vi "Play Cine from File.vi"() -> ()   [LabVIEW 2013]
doc: "This example VI demonstrates how to acquire and display captured images stored in the internal RAM of a Phantom Camera using the Vision Research Phantom Series LabVIEW Driver."
uses:
  _Type Defs/PhFile InfName.ctl
  _Type Defs/PHCon IMRANGE.ctl
  _Type Defs/PhInt PhProcessImage Selectors.ctl
  VRI.lvlib
panel:
  in  "Delay (ms)":u32=100
  in  "szFileName":path
  in  "fGain16_8":dbl=1.0
  in  "Stop":bool
  out "Image Count":u32
  out "first image number":i32
  out "Current Image #":i32
  out "Preview":picture
  out "Error Out":errorcluster
  in  "error in (no error)":errorcluster
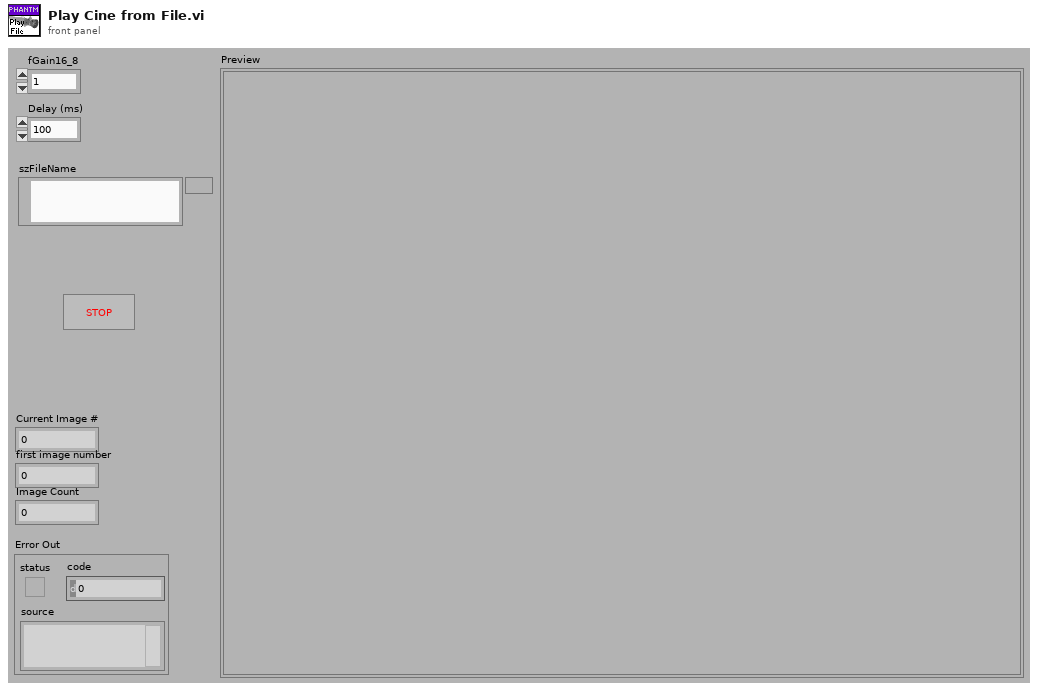
[diagram p1: front panel]
types:
  T1 = typedef "VRI.lvlib/PHCon IMRANGE.ctl" = cluster{"First":i32, "Cnt":u32}
  T2 = typedef "VRI.lvlib/PhFile InfName.ctl" = u32
  T3 = typedef "VRI.lvlib/PhInt PhProcessImage Selectors.ctl" = u16
  T4 = typedef "VRI.lvlib/PhInt IH.ctl" = cluster{"biSize":u32, "biWidth":i32, "biHeight":i32, "biPlanes":u16, "biBitCount":u16, "biCompresssion":u32, "biSizeImage":u32, "biXPelsPerMeter":i32, "biYPelsPerMeter":i32, "biClrUsed":u32, "biClrImportant":u32, "BlackLevel":i32, "WhiteLevel":i32}
  T5 = typedef "VRI.lvlib/BITMAPINFOHEADER.ctl" = cluster{"biSize":u32, "biWidth":i32, "biHeight":i32, "biPlanes":u16, "biBitCount":u16, "biCompression":u32, "biSizeImage":u32, "biXPelsPerMeter":i32, "biYPelsPerMeter":i32, "biClrUsed":u32, "biClrImportant":u32}
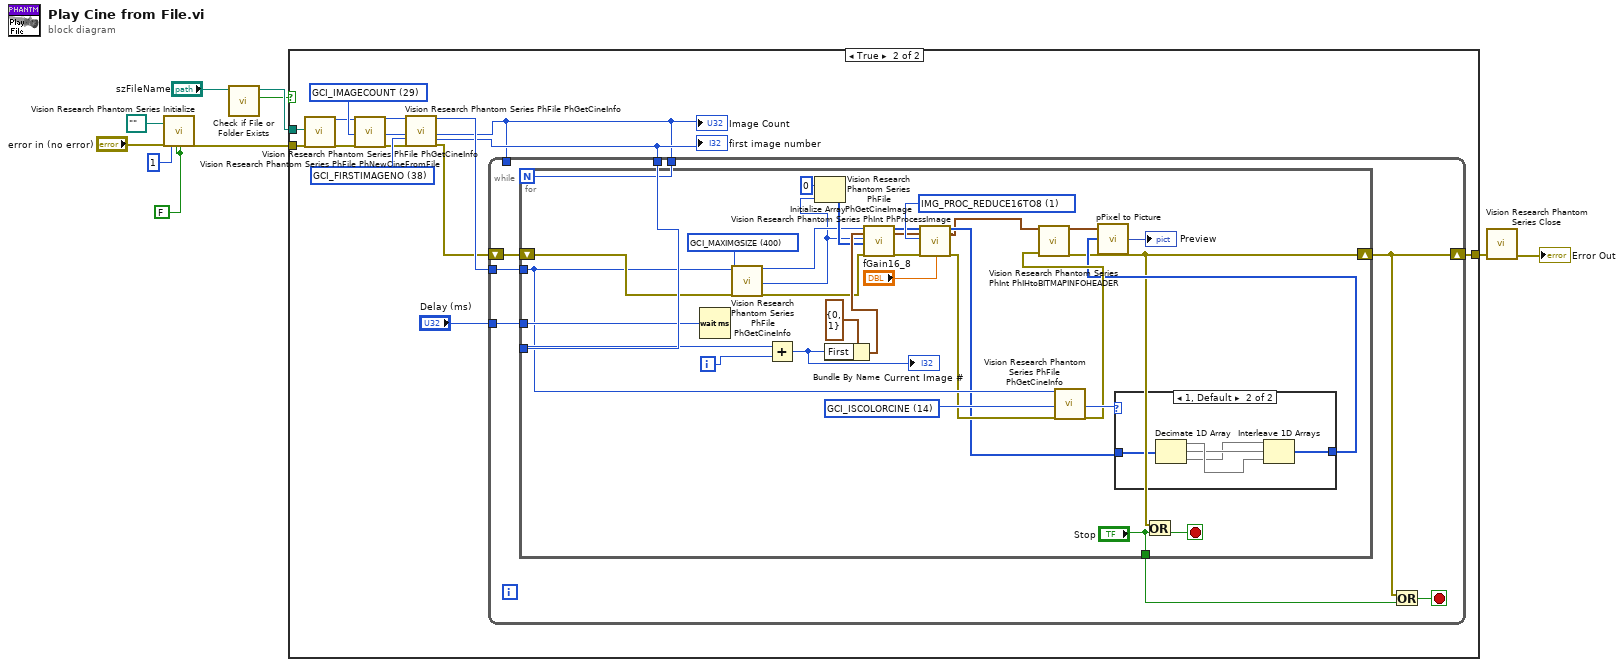
[diagram p0: block diagram]
diagram:
  w7 = FALSE ("ID Query (T: Check)")
  n1 = call "Vision Research Phantom Series Initialize.vi"("Storage Path (\"\")"=path "" ("Storage Path (\"\")"), "error in (no error)"="error in (no error)", "CallID"=u32 1, "ID Query (T: Check)"=w7, "Reset (F: Don't Reset)"=w7) -> ("Error Out"=w4:errorcluster)  [unwired: 14 out]
  n2 = call <vilib>:"Check if File or Folder Exists.vi"("path"="szFileName") -> ("file or folder exists?"=w1:bool, "dup path"=w2:path)  [unwired: 8 in, 1 out]
  n3 = case shown="True" w1 {
    tunnel: [w11 w25] -> w6
    tunnel: w2 -> [_ w24]
    tunnel: w4 -> [w11 w22]
    frame False {
    }
    frame True {
      w18 = T2 38 items=["GCI_CFA"=0, "GCI_FRAMERATE"=1, "GCI_EXPOSURE"=2, "GCI_AUTOEXPOSURE"=3, "GCI_REALBPP"=4, "GCI_CAMERASERIAL"=5, "GCI_HEADSERIAL0"=6, "GCI_HEADSERIAL1"=7, "GCI_HEADSERIAL2"=8, "GCI_HEADSERIAL3"=9, "GCI_TRIGTIMESEC"=10, "GCI_TRIGTIMEFR"=11, "GCI_ISFILECINE"=12, "GCI_IS16BPPCINE"=13, "GCI_ISCOLORCINE"=14, "GCI_ISMULTIHEADCINE"=15, "GCI_EXPOSURENS"=16, "GCI_EDREXPOSURENS"=17, "GCI_FRAMEDELAYNS"=19, "GCI_FROMFILETYPE"=20, "GCI_COMPRESSION"=21, "GCI_CAMERAVERSION"=22, "GCI_ROTATE"=23, "GCI_IMWIDTH"=24, "GCI_IMHEIGHT"=25, "GCI_IMWIDTHACQ"=26, "GCI_IMHEIGHTACQ"=27, "GCI_POSTTRIGGER"=28, "GCI_IMAGECOUNT"=29, "GCI_TOTALIMAGECOUNT"=30, "GCI_TRIGFRAME"=31, "GCI_AUTOEXPLEVEL"=32, "GCI_AUTOEXPTOP"=33, "GCI_AUTOEXPLEFT"=34, "GCI_AUTOEXPBOTTOM"=35, "GCI_AUTOEXPRIGHT"=36, "GCI_RECORDINGTIMEZONE"=37, "GCI_FIRSTIMAGENO"=38, "GCI_FIRSTMOVIEIMAGE"=39, "GCI_CINENAME"=40, "GCI_FRPSTEPS"=100, "GCI_FRP1X"=101, "GCI_FRP1Y"=102, "GCI_FRP2X"=103, "GCI_FRP2Y"=104, "GCI_FRP3X"=105, "GCI_FRP3Y"=106, "GCI_FRP4X"=107, "GCI_FRP4Y"=108, "GCI_WRITEERR"=109, "GCI_LENSDESCRIPTION"=110, "GCI_LENSAPERATURE"=111, "GCI_LENSFOCALLENGTH"=112, "GCI_WB"=200, "GCI_WBVIEW"=201, "GCI_BRIGHT"=202, "GCI_CONTRAST"=203, "GCI_GAMMA"=204, "GCI_GAMMAR"=223, "GCI_GAMMAB"=224, "GCI_SATURATION"=205, "GCI_HUE"=206, "GCI_FLIPH"=207, "GCI_FLIPV"=208, "GCI_FILTERCODE"=209, "GCI_IMFILTER"=210, "GCI_INTALGO"=211, "GCI_PEDESTALR"=212, "GCI_PEDESTALG"=213, "GCI_PEDESTALB"=214, "GCI_FLARE"=225, "GCI_CHROMA"=226, "GCI_TONE"=227, "GCI_ENABLEMATRICES"=228, "GCI_USERMATRIX"=229, "GCI_RESAMPLEACTIVE"=215, "GCI_RESAMPLEWIDTH"=216, "GCI_RESAMPLEHEIGHT"=217, "GCI_CROPACTIVE"=218, "GCI_CROPRECTANGLE"=219, "GCI_OFFSET16_8"=220, "GCI_GAIN16_8"=221, "GCI_DEMOSAICINGFUNCPTR"=222, "GCI_VFLIPVIEWACTIVE"=300, "GCI_MAXIMGSIZE"=400, "GCI_FRPIMGNOARRAY"=450, "GCI_FRPRATEARRAY"=451, "GCI_FRPSHAPEARRAY"=452, "GCI_TRIGTC"=470, "GCI_TRIGTCU"=471, "GCI_PBRATE"=472, "GCI_TCRATE"=473, "GCI_SAVERANGE"=500, "GCI_SAVEFILENAME"=501, "GCI_SAVEFILETYPE"=502, "GCI_SAVE16BIT"=503, "GCI_SAVEPACKED"=504, "GCI_SAVEXML"=505, "GCI_SAVESTAMPTIME"=506, "GCI_SAVEAVIFRAMERATE"=520, "GCI_SAVEAVICOMPRESSORLIST"=521, "GCI_SAVEAVICOMPRESSORINDEX"=522, "GCI_SAVEDPXLSB"=530, "GCI_SAVEDPXTO10BPS"=531, "GCI_SAVEDPXDATAPACKING"=532, "GCI_SAVEDPX10BITLOG"=533, "GCI_SAVEDPXEXPORTLOGLUT"=534, "GCI_SAVEDPX10BITLOGREFWHITE"=535, "GCI_SAVEDPX10BITLOGREFBLACK"=536, "GCI_SAVEDPX10BITLOGGAMMA"=537, "GCI_SAVEDPX10BITLOGFILMGAMMA"=538, "GCI_SAVEQTPLAYBACKRATE"=550, "GCI_SAVECCIQUALITY"=560, "GCI_UNCALIBRATEDIMAGE"=600, "GCI_NOPROCESSING"=601, "GCI_BADPIXELREPAIR"=602] ("InfName")
      w21 = T2 29 items=["GCI_CFA"=0, "GCI_FRAMERATE"=1, "GCI_EXPOSURE"=2, "GCI_AUTOEXPOSURE"=3, "GCI_REALBPP"=4, "GCI_CAMERASERIAL"=5, "GCI_HEADSERIAL0"=6, "GCI_HEADSERIAL1"=7, "GCI_HEADSERIAL2"=8, "GCI_HEADSERIAL3"=9, "GCI_TRIGTIMESEC"=10, "GCI_TRIGTIMEFR"=11, "GCI_ISFILECINE"=12, "GCI_IS16BPPCINE"=13, "GCI_ISCOLORCINE"=14, "GCI_ISMULTIHEADCINE"=15, "GCI_EXPOSURENS"=16, "GCI_EDREXPOSURENS"=17, "GCI_FRAMEDELAYNS"=19, "GCI_FROMFILETYPE"=20, "GCI_COMPRESSION"=21, "GCI_CAMERAVERSION"=22, "GCI_ROTATE"=23, "GCI_IMWIDTH"=24, "GCI_IMHEIGHT"=25, "GCI_IMWIDTHACQ"=26, "GCI_IMHEIGHTACQ"=27, "GCI_POSTTRIGGER"=28, "GCI_IMAGECOUNT"=29, "GCI_TOTALIMAGECOUNT"=30, "GCI_TRIGFRAME"=31, "GCI_AUTOEXPLEVEL"=32, "GCI_AUTOEXPTOP"=33, "GCI_AUTOEXPLEFT"=34, "GCI_AUTOEXPBOTTOM"=35, "GCI_AUTOEXPRIGHT"=36, "GCI_RECORDINGTIMEZONE"=37, "GCI_FIRSTIMAGENO"=38, "GCI_FIRSTMOVIEIMAGE"=39, "GCI_CINENAME"=40, "GCI_FRPSTEPS"=100, "GCI_FRP1X"=101, "GCI_FRP1Y"=102, "GCI_FRP2X"=103, "GCI_FRP2Y"=104, "GCI_FRP3X"=105, "GCI_FRP3Y"=106, "GCI_FRP4X"=107, "GCI_FRP4Y"=108, "GCI_WRITEERR"=109, "GCI_LENSDESCRIPTION"=110, "GCI_LENSAPERATURE"=111, "GCI_LENSFOCALLENGTH"=112, "GCI_WB"=200, "GCI_WBVIEW"=201, "GCI_BRIGHT"=202, "GCI_CONTRAST"=203, "GCI_GAMMA"=204, "GCI_GAMMAR"=223, "GCI_GAMMAB"=224, "GCI_SATURATION"=205, "GCI_HUE"=206, "GCI_FLIPH"=207, "GCI_FLIPV"=208, "GCI_FILTERCODE"=209, "GCI_IMFILTER"=210, "GCI_INTALGO"=211, "GCI_PEDESTALR"=212, "GCI_PEDESTALG"=213, "GCI_PEDESTALB"=214, "GCI_FLARE"=225, "GCI_CHROMA"=226, "GCI_TONE"=227, "GCI_ENABLEMATRICES"=228, "GCI_USERMATRIX"=229, "GCI_RESAMPLEACTIVE"=215, "GCI_RESAMPLEWIDTH"=216, "GCI_RESAMPLEHEIGHT"=217, "GCI_CROPACTIVE"=218, "GCI_CROPRECTANGLE"=219, "GCI_OFFSET16_8"=220, "GCI_GAIN16_8"=221, "GCI_DEMOSAICINGFUNCPTR"=222, "GCI_VFLIPVIEWACTIVE"=300, "GCI_MAXIMGSIZE"=400, "GCI_FRPIMGNOARRAY"=450, "GCI_FRPRATEARRAY"=451, "GCI_FRPSHAPEARRAY"=452, "GCI_TRIGTC"=470, "GCI_TRIGTCU"=471, "GCI_PBRATE"=472, "GCI_TCRATE"=473, "GCI_SAVERANGE"=500, "GCI_SAVEFILENAME"=501, "GCI_SAVEFILETYPE"=502, "GCI_SAVE16BIT"=503, "GCI_SAVEPACKED"=504, "GCI_SAVEXML"=505, "GCI_SAVESTAMPTIME"=506, "GCI_SAVEAVIFRAMERATE"=520, "GCI_SAVEAVICOMPRESSORLIST"=521, "GCI_SAVEAVICOMPRESSORINDEX"=522, "GCI_SAVEDPXLSB"=530, "GCI_SAVEDPXTO10BPS"=531, "GCI_SAVEDPXDATAPACKING"=532, "GCI_SAVEDPX10BITLOG"=533, "GCI_SAVEDPXEXPORTLOGLUT"=534, "GCI_SAVEDPX10BITLOGREFWHITE"=535, "GCI_SAVEDPX10BITLOGREFBLACK"=536, "GCI_SAVEDPX10BITLOGGAMMA"=537, "GCI_SAVEDPX10BITLOGFILMGAMMA"=538, "GCI_SAVEQTPLAYBACKRATE"=550, "GCI_SAVECCIQUALITY"=560, "GCI_UNCALIBRATEDIMAGE"=600, "GCI_NOPROCESSING"=601, "GCI_BADPIXELREPAIR"=602] ("InfName")
      n4 = call "Vision Research Phantom Series PhFile PhNewCineFromFile.vi"("szFileName"=w24, "Error In (no error)"=w22) -> ("pCH"=w19:u32, "Error Out"=w20:errorcluster)  [unwired: 1 in, 15 out]
      n5 = call "Vision Research Phantom Series PhFile PhGetCineInfo.vi"("CH in"=w19, "InfName"=w21, "Error In (no error)"=w20) -> ("CH out"=w16:u32, "pInfVal out"=w12:i32, "Error Out"=w17:errorcluster)  [unwired: 14 in]
      "Image Count" <- w12
      n6 = call "Vision Research Phantom Series PhFile PhGetCineInfo.vi"("CH in"=w16, "InfName"=w18, "Error In (no error)"=w17) -> ("CH out"=w15:u32, "pInfVal out"=w13:i32, "Error Out"=w14:errorcluster)  [unwired: 14 in]
      "first image number" <- w13
      n7 = while {
        tunnel: w13 -> [w32]
        tunnel: w12 -> [w28]
        tunnel: w12 -> [_]
        tunnel: w15 -> [w30]
        tunnel: "Delay (ms)" -> [w29]
        shift-right: [w26] -> w25
        shift-left: w14 -> [w33]
        stop <- w27 stop-if-true
        n8 = for {
          N: w28 -> [_]
          tunnel: w32 -> [w59]
          tunnel: ["Stop"] -> w31
          tunnel: w30 -> [w41]
          tunnel: w29 -> [w45]
          shift-right: [w34] -> w26
          shift-left: w33 -> [w49]
          i -> [w63]
          stop <- w35 stop-if-true
          w43 = T2 14 items=["GCI_CFA"=0, "GCI_FRAMERATE"=1, "GCI_EXPOSURE"=2, "GCI_AUTOEXPOSURE"=3, "GCI_REALBPP"=4, "GCI_CAMERASERIAL"=5, "GCI_HEADSERIAL0"=6, "GCI_HEADSERIAL1"=7, "GCI_HEADSERIAL2"=8, "GCI_HEADSERIAL3"=9, "GCI_TRIGTIMESEC"=10, "GCI_TRIGTIMEFR"=11, "GCI_ISFILECINE"=12, "GCI_IS16BPPCINE"=13, "GCI_ISCOLORCINE"=14, "GCI_ISMULTIHEADCINE"=15, "GCI_EXPOSURENS"=16, "GCI_EDREXPOSURENS"=17, "GCI_FRAMEDELAYNS"=19, "GCI_FROMFILETYPE"=20, "GCI_COMPRESSION"=21, "GCI_CAMERAVERSION"=22, "GCI_ROTATE"=23, "GCI_IMWIDTH"=24, "GCI_IMHEIGHT"=25, "GCI_IMWIDTHACQ"=26, "GCI_IMHEIGHTACQ"=27, "GCI_POSTTRIGGER"=28, "GCI_IMAGECOUNT"=29, "GCI_TOTALIMAGECOUNT"=30, "GCI_TRIGFRAME"=31, "GCI_AUTOEXPLEVEL"=32, "GCI_AUTOEXPTOP"=33, "GCI_AUTOEXPLEFT"=34, "GCI_AUTOEXPBOTTOM"=35, "GCI_AUTOEXPRIGHT"=36, "GCI_RECORDINGTIMEZONE"=37, "GCI_FIRSTIMAGENO"=38, "GCI_FIRSTMOVIEIMAGE"=39, "GCI_CINENAME"=40, "GCI_FRPSTEPS"=100, "GCI_FRP1X"=101, "GCI_FRP1Y"=102, "GCI_FRP2X"=103, "GCI_FRP2Y"=104, "GCI_FRP3X"=105, "GCI_FRP3Y"=106, "GCI_FRP4X"=107, "GCI_FRP4Y"=108, "GCI_WRITEERR"=109, "GCI_LENSDESCRIPTION"=110, "GCI_LENSAPERATURE"=111, "GCI_LENSFOCALLENGTH"=112, "GCI_WB"=200, "GCI_WBVIEW"=201, "GCI_BRIGHT"=202, "GCI_CONTRAST"=203, "GCI_GAMMA"=204, "GCI_GAMMAR"=223, "GCI_GAMMAB"=224, "GCI_SATURATION"=205, "GCI_HUE"=206, "GCI_FLIPH"=207, "GCI_FLIPV"=208, "GCI_FILTERCODE"=209, "GCI_IMFILTER"=210, "GCI_INTALGO"=211, "GCI_PEDESTALR"=212, "GCI_PEDESTALG"=213, "GCI_PEDESTALB"=214, "GCI_FLARE"=225, "GCI_CHROMA"=226, "GCI_TONE"=227, "GCI_ENABLEMATRICES"=228, "GCI_USERMATRIX"=229, "GCI_RESAMPLEACTIVE"=215, "GCI_RESAMPLEWIDTH"=216, "GCI_RESAMPLEHEIGHT"=217, "GCI_CROPACTIVE"=218, "GCI_CROPRECTANGLE"=219, "GCI_OFFSET16_8"=220, "GCI_GAIN16_8"=221, "GCI_DEMOSAICINGFUNCPTR"=222, "GCI_VFLIPVIEWACTIVE"=300, "GCI_MAXIMGSIZE"=400, "GCI_FRPIMGNOARRAY"=450, "GCI_FRPRATEARRAY"=451, "GCI_FRPSHAPEARRAY"=452, "GCI_TRIGTC"=470, "GCI_TRIGTCU"=471, "GCI_PBRATE"=472, "GCI_TCRATE"=473, "GCI_SAVERANGE"=500, "GCI_SAVEFILENAME"=501, "GCI_SAVEFILETYPE"=502, "GCI_SAVE16BIT"=503, "GCI_SAVEPACKED"=504, "GCI_SAVEXML"=505, "GCI_SAVESTAMPTIME"=506, "GCI_SAVEAVIFRAMERATE"=520, "GCI_SAVEAVICOMPRESSORLIST"=521, "GCI_SAVEAVICOMPRESSORINDEX"=522, "GCI_SAVEDPXLSB"=530, "GCI_SAVEDPXTO10BPS"=531, "GCI_SAVEDPXDATAPACKING"=532, "GCI_SAVEDPX10BITLOG"=533, "GCI_SAVEDPXEXPORTLOGLUT"=534, "GCI_SAVEDPX10BITLOGREFWHITE"=535, "GCI_SAVEDPX10BITLOGREFBLACK"=536, "GCI_SAVEDPX10BITLOGGAMMA"=537, "GCI_SAVEDPX10BITLOGFILMGAMMA"=538, "GCI_SAVEQTPLAYBACKRATE"=550, "GCI_SAVECCIQUALITY"=560, "GCI_UNCALIBRATEDIMAGE"=600, "GCI_NOPROCESSING"=601, "GCI_BADPIXELREPAIR"=602] ("InfName")
          w46 = T2 400 items=["GCI_CFA"=0, "GCI_FRAMERATE"=1, "GCI_EXPOSURE"=2, "GCI_AUTOEXPOSURE"=3, "GCI_REALBPP"=4, "GCI_CAMERASERIAL"=5, "GCI_HEADSERIAL0"=6, "GCI_HEADSERIAL1"=7, "GCI_HEADSERIAL2"=8, "GCI_HEADSERIAL3"=9, "GCI_TRIGTIMESEC"=10, "GCI_TRIGTIMEFR"=11, "GCI_ISFILECINE"=12, "GCI_IS16BPPCINE"=13, "GCI_ISCOLORCINE"=14, "GCI_ISMULTIHEADCINE"=15, "GCI_EXPOSURENS"=16, "GCI_EDREXPOSURENS"=17, "GCI_FRAMEDELAYNS"=19, "GCI_FROMFILETYPE"=20, "GCI_COMPRESSION"=21, "GCI_CAMERAVERSION"=22, "GCI_ROTATE"=23, "GCI_IMWIDTH"=24, "GCI_IMHEIGHT"=25, "GCI_IMWIDTHACQ"=26, "GCI_IMHEIGHTACQ"=27, "GCI_POSTTRIGGER"=28, "GCI_IMAGECOUNT"=29, "GCI_TOTALIMAGECOUNT"=30, "GCI_TRIGFRAME"=31, "GCI_AUTOEXPLEVEL"=32, "GCI_AUTOEXPTOP"=33, "GCI_AUTOEXPLEFT"=34, "GCI_AUTOEXPBOTTOM"=35, "GCI_AUTOEXPRIGHT"=36, "GCI_RECORDINGTIMEZONE"=37, "GCI_FIRSTIMAGENO"=38, "GCI_FIRSTMOVIEIMAGE"=39, "GCI_CINENAME"=40, "GCI_FRPSTEPS"=100, "GCI_FRP1X"=101, "GCI_FRP1Y"=102, "GCI_FRP2X"=103, "GCI_FRP2Y"=104, "GCI_FRP3X"=105, "GCI_FRP3Y"=106, "GCI_FRP4X"=107, "GCI_FRP4Y"=108, "GCI_WRITEERR"=109, "GCI_LENSDESCRIPTION"=110, "GCI_LENSAPERATURE"=111, "GCI_LENSFOCALLENGTH"=112, "GCI_WB"=200, "GCI_WBVIEW"=201, "GCI_BRIGHT"=202, "GCI_CONTRAST"=203, "GCI_GAMMA"=204, "GCI_GAMMAR"=223, "GCI_GAMMAB"=224, "GCI_SATURATION"=205, "GCI_HUE"=206, "GCI_FLIPH"=207, "GCI_FLIPV"=208, "GCI_FILTERCODE"=209, "GCI_IMFILTER"=210, "GCI_INTALGO"=211, "GCI_PEDESTALR"=212, "GCI_PEDESTALG"=213, "GCI_PEDESTALB"=214, "GCI_FLARE"=225, "GCI_CHROMA"=226, "GCI_TONE"=227, "GCI_ENABLEMATRICES"=228, "GCI_USERMATRIX"=229, "GCI_RESAMPLEACTIVE"=215, "GCI_RESAMPLEWIDTH"=216, "GCI_RESAMPLEHEIGHT"=217, "GCI_CROPACTIVE"=218, "GCI_CROPRECTANGLE"=219, "GCI_OFFSET16_8"=220, "GCI_GAIN16_8"=221, "GCI_DEMOSAICINGFUNCPTR"=222, "GCI_VFLIPVIEWACTIVE"=300, "GCI_MAXIMGSIZE"=400, "GCI_FRPIMGNOARRAY"=450, "GCI_FRPRATEARRAY"=451, "GCI_FRPSHAPEARRAY"=452, "GCI_TRIGTC"=470, "GCI_TRIGTCU"=471, "GCI_PBRATE"=472, "GCI_TCRATE"=473, "GCI_SAVERANGE"=500, "GCI_SAVEFILENAME"=501, "GCI_SAVEFILETYPE"=502, "GCI_SAVE16BIT"=503, "GCI_SAVEPACKED"=504, "GCI_SAVEXML"=505, "GCI_SAVESTAMPTIME"=506, "GCI_SAVEAVIFRAMERATE"=520, "GCI_SAVEAVICOMPRESSORLIST"=521, "GCI_SAVEAVICOMPRESSORINDEX"=522, "GCI_SAVEDPXLSB"=530, "GCI_SAVEDPXTO10BPS"=531, "GCI_SAVEDPXDATAPACKING"=532, "GCI_SAVEDPX10BITLOG"=533, "GCI_SAVEDPXEXPORTLOGLUT"=534, "GCI_SAVEDPX10BITLOGREFWHITE"=535, "GCI_SAVEDPX10BITLOGREFBLACK"=536, "GCI_SAVEDPX10BITLOGGAMMA"=537, "GCI_SAVEDPX10BITLOGFILMGAMMA"=538, "GCI_SAVEQTPLAYBACKRATE"=550, "GCI_SAVECCIQUALITY"=560, "GCI_UNCALIBRATEDIMAGE"=600, "GCI_NOPROCESSING"=601, "GCI_BADPIXELREPAIR"=602] ("InfName")
          w54 = T3 1 items=["IMG_PROC_REDUCE16TO8"=1] ("procID")
          n9 = Wait (ms)(milliseconds to wait=w45) -> ()  [unwired: 1 out]
          n10 = call "Vision Research Phantom Series PhFile PhGetCineInfo.vi"("CH in"=w41, "InfName"=w46, "Error In (no error)"=w49) -> ("CH out"=w47:u32, "pInfVal out"=w44:i32, "Error Out"=w48:errorcluster)  [unwired: 14 in]
          n11 = Add(x=w59, y=w63) -> (x+y=w60:i32)
          "Current Image #" <- w60
          n12 = Initialize Array(u16 0 ("element"), w44) -> (w56:u16[])
          n13 = Bundle By Name(cluster=T1 {"First"=0, "Cnt"=1} ("pRng"), "First"=w60) -> (w57:T1)
          n14 = call "Vision Research Phantom Series PhFile PhGetCineImage.vi"("hC [in]"=w47, "pRng [in]"=w57, "bufferByteSize [in]"=w44, "pPixelBuffer [in]"=w56, "Error In (no error)"=w48) -> ("pPixelBuffer [out]"=w52:u16[], "IH [out]"=w51:T4, "Error Out"=w50:errorcluster)  [unwired: 11 in, 1 out]
          n15 = call "Vision Research Phantom Series PhInt PhProcessImage.vi"("pPixelSrc [in]"=w52, "IH [in]"=w51, "procID"=w54, "pProcParams"="fGain16_8", "Error In (no error)"=w50) -> ("pPixelDest [out]"=w38:u8[], "IH [out]"=w36:T4, "Error Out"=w40:errorcluster)  [unwired: 12 in]
          n16 = call "Vision Research Phantom Series PhFile PhGetCineInfo.vi"("CH in"=w41, "InfName"=w43, "Error In (no error)"=w40) -> ("pInfVal out"=w42:i32, "Error Out"=w39:errorcluster)  [unwired: 15 out]
          n17 = call "Vision Research Phantom Series PhInt PhIHtoBITMAPINFOHEADER.vi"("IH"=w36, "Error In (no error)"=w39) -> ("BITMAPINFOHEADER"=w55:T5, "Error Out"=w34:errorcluster)  [unwired: 16 in]
          n18 = case shown="1, Default" w42 {
            tunnel: [w65 w67] -> w37
            tunnel: w38 -> [w65 w66]
            frame 0 {
            }
            frame 1, Default {
              n19 = Decimate 1D Array(w66) -> (w70:u8[], w69:u8[], w68:u8[])
              n20 = Interleave 1D Arrays(w68, w69, w70) -> (w67:u8[])
            }
          }
          n21 = call "pPixel to Picture.vi"("pPixel"=w37, "BITMAPINFOHEADER"=w55) -> ("Preview"=→"Preview":picture)  [unwired: 1 in]
          n22 = Or(x=w34, y="Stop") -> (x .or. y?=w35:bool)
        }
        n23 = Or(x=w26, y=w31) -> (x .or. y?=w27:bool)
      }
    }
  }
  n24 = call "Vision Research Phantom Series Close.vi"("Error In (no error)"=w6) -> ("Error Out"=→"Error Out":errorcluster)  [unwired: 18 out]
